vi "阀配置写入.vi"(8 "error in (no error)":errorcluster caption="错误输入（无错误）", 10 "data":T1 {"Value" items=["三通阀", "排阀"]}, 11 "SingleStepTestV3 输入":refnum<class "SingleStepCODMnV2.lvclass">) -> (0 "error out":errorcluster caption="错误输出", 3 "SingleStepTestV3 输出":refnum<class "SingleStepCODMnV2.lvclass">)   [LabVIEW 2022 SP3, in "SingleStepCODMnV2.lvlib" / "SingleStepCODMnV2.lvclass"]
uses:
  SingleStepCODMnV2.lvclass
  SingleStepCODMnV2.lvclass/SingleStepCODMnV2.ctl
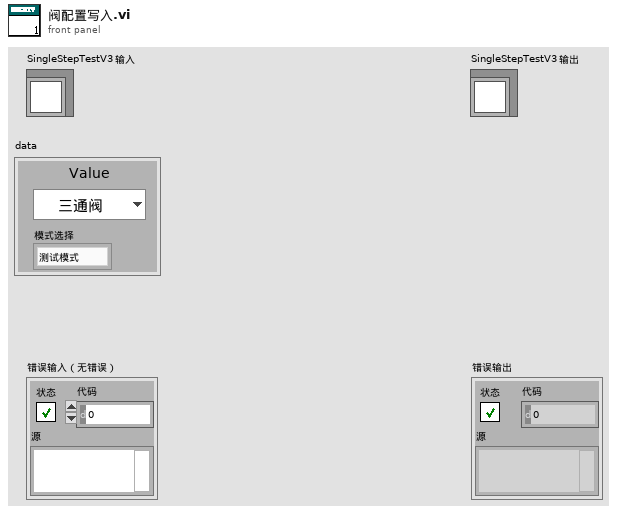
[diagram p1: front panel]
types:
  T1 = cluster{"Value":u8, "模式选择":enum16{"测试模式", "流程模式"}}
  T2 = enum8{"Enabled", "Disabled", "Disabled and Grayed Out"}
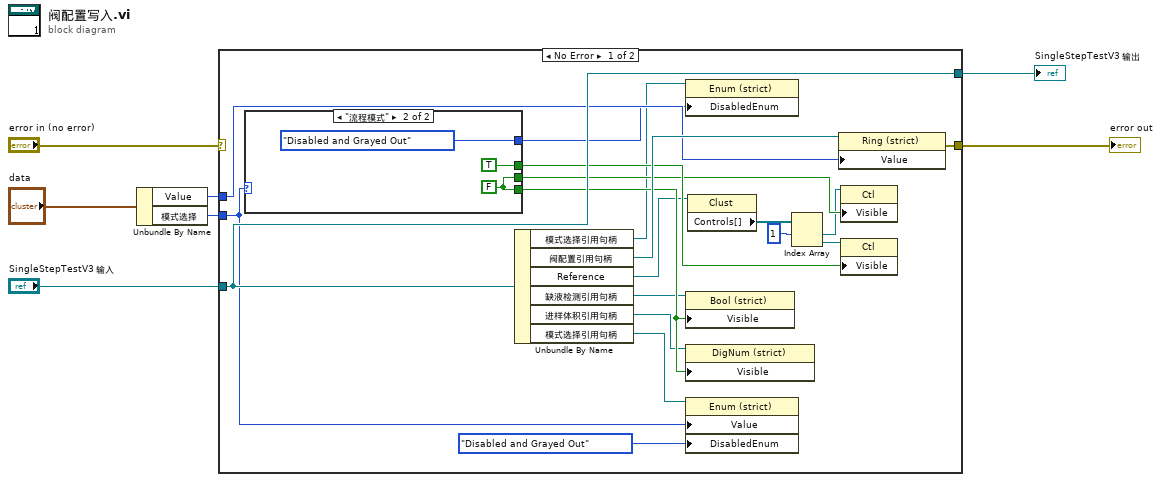
[diagram p0: block diagram]
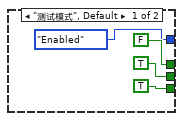
[diagram p2: hidden frame]
diagram:
  n1 = Unbundle By Name("data") -> ("Value"=w2:u8, "模式选择"=w1:enum16{"测试模式", "流程模式"})
  n2 = case shown="No Error" "error in (no error)" {
    selector: "error in (no error)" -> [_ w35]
    tunnel: [w24 w35] -> w6
    tunnel: [w25 w34] -> w4
    tunnel: "SingleStepTestV3 输入" -> [w25 w34]
    tunnel: w2 -> [w11 _]
    tunnel: w1 -> [w10 _]
    frame No Error {
      n3 = case shown="\"流程模式\"" w10 {
        tunnel: [TRUE w32] -> w21
        tunnel: [FALSE TRUE] -> w22
        tunnel: [TRUE ("可见") w32] -> w23
        tunnel: [T2."Enabled" ("禁用") T2."Disabled and Grayed Out" ("禁用")] -> w8
        frame "测试模式", Default {
        }
        frame "流程模式" {
          w32 = FALSE
        }
      }
      n4 = Unbundle By Name(w25) -> ("模式选择引用句柄"=w9:refnum<vi>, "阀配置引用句柄"=w26:refnum<vi>, "Reference"=w16:refnum<vi>, "缺液检测引用句柄"=w15:refnum<vi>, "进样体积引用句柄"=w14:refnum<vi>, "模式选择引用句柄"=w13:refnum<vi>)
      n5 = property class="Enum (strict)"(reference=w9, "DisabledEnum"=w8) -> ()  [unwired: 1 in, 2 out]
      n6 = property class="Bool (strict)"(reference=w15, "Visible"=w23) -> ()  [unwired: 1 in, 2 out]
      n7 = property class="DigNum (strict)"(reference=w14, "Visible"=w23) -> ()  [unwired: 1 in, 2 out]
      n8 = property class="Enum (strict)"(reference=w13, "Value"=w10, "DisabledEnum"=T2."Disabled and Grayed Out" ("禁用")) -> ()  [unwired: 1 in, 2 out]
      n9 = property class="Clust"(reference=w16) -> ("Controls[]"=w18:refnum<vi>[])  [unwired: 1 in, 2 out]
      n10 = Index Array(array=w18, index #1=1 ("索引")) -> (element #1=w19:refnum<vi>, element #2=w20:refnum<vi>)  [unwired: 1 in]
      n11 = property class="Ring (strict)"(reference=w26, "Value"=w11) -> (error out=w24:errorcluster)  [unwired: 1 in, 1 out]
      n12 = property class="Ctl"(reference=w19, "Visible"=w21) -> ()  [unwired: 1 in, 2 out]
      n13 = property class="Ctl"(reference=w20, "Visible"=w22) -> ()  [unwired: 1 in, 2 out]
    }
    frame Error {
    }
  }
  "error out" <- w6
  "SingleStepTestV3 输出" <- w4
